vi "DataTypeAssignment.vi"() -> ()   [LabVIEW 2019]
panel:
  out "BoolInd":bool
  in  "BoolCtrl":bool
  out "StrInd":string
  in  "StrCtrl":string
  out "bInd":u8
  in  "bCtrl":u8
  out "aInd":dbl
  in  "aCtrl":dbl
  # "Indicator"
  # "Control"
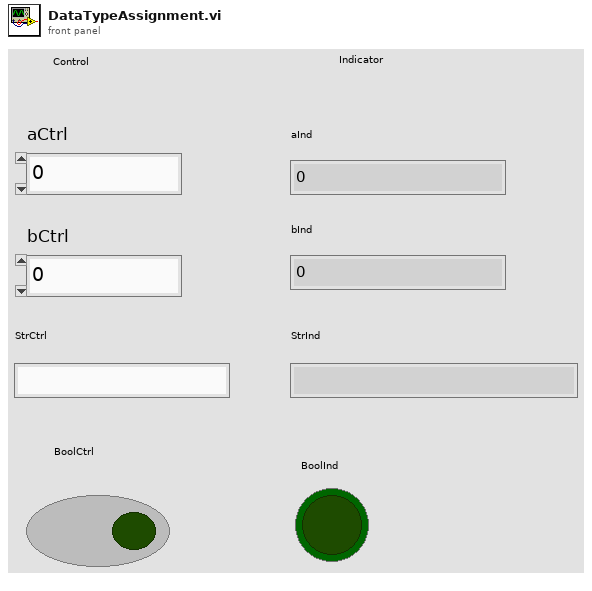
[diagram p1: front panel]
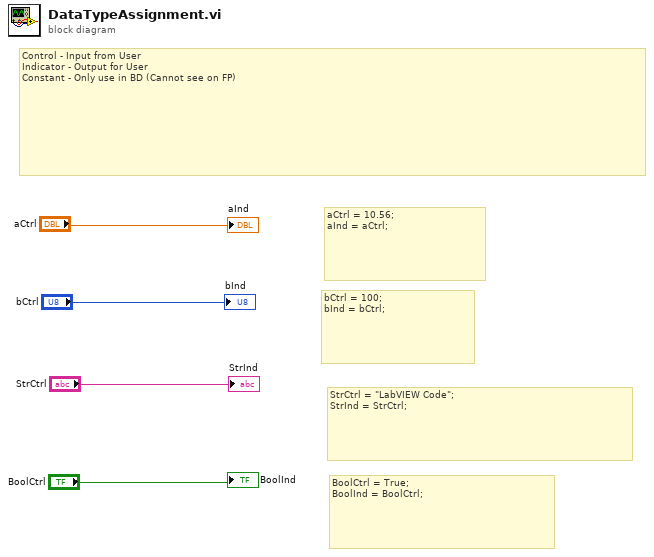
[diagram p0: block diagram]
diagram:
  # "BoolCtrl = True;\nBoolInd = BoolCtrl;"
  # "StrCtrl = \"LabVIEW Code\";\nStrInd = StrCtrl;"
  # "bCtrl = 100;\nbInd = bCtrl;"
  # "aCtrl = 10.56;\naInd = aCtrl;"
  # "Control - Input from User \nIndicator - Output for User\nConstant - Only use in BD (Cannot see on FP)"
  "aInd" <- "aCtrl"
  "bInd" <- "bCtrl"
  "StrInd" <- "StrCtrl"
  "BoolInd" <- "BoolCtrl"
